vi "Initialize Dialog.vi"(8 "error in (no error)":errorcluster, 9 "SubPnl Refnum":refnum<vi>, 10 "VI Refnum":refnum<vi>, 11 "DataGrid Config Dialog in":refnum<class "DataGrid Config Dialog.lvclass">) -> (0 "error out":errorcluster, 1 "Data Type Selector Return":refnum<user-event>, 2 "Return Data":refnum<user-event>, 3 "DataGrid Config Dialog out":refnum<class "DataGrid Config Dialog.lvclass">)   [LabVIEW 2018, in "DataGrid Config Dialog.lvclass"]
uses:
  DataGrid Config Dialog.lvclass
  Data Type Classes/Generic/Generic Data Type.lvclass
  <vilib>/MGI/Panel Manager/Panel/Panel/Window/Dialog/Behavior.ctl
  DataGrid Config Dialog.lvclass/DataGrid Config Dialog.ctl
  <vilib>/MGI/Panel Manager/Panel/Panel/Subpanel/Subpanel.lvclass
  C:/Program Files (x86)/National Instruments/LabVIEW 2018/vi.lib/MGI/Panel Manager/Panel/Panel/Panel.lvclass
  <vilib>/MGI/Panel Manager/Panel/Panel/Window/Dialog/Dialog.lvclass
  <vilib>/MGI/Panel Manager/Panel/Panel/Subpanel/Subpanel.vi
  <vilib>/MGI/Panel Manager/Panel/Panel/Window/Dialog/Dialog.vi
  <vilib>/MGI/Panel Manager/Panel/Panel.lvlib
  <vilib>/MGI/Panel Manager/Panel/Panel/Panel.lvclass
  DataGrid Config/DataGrid Config.lvclass
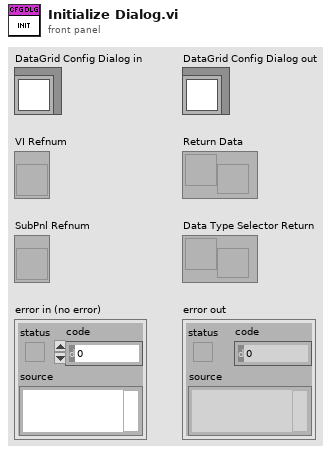
[diagram p1: front panel]
types:
  T1 = enum8{"Enabled", "Disabled", "Disabled and Grayed Out"}
  T2 = typedef "Panel.lvlib/Dialog.lvclass/Behavior.ctl" = enum32{"Floating", "Floating/Auto-Hide", "Modal"}
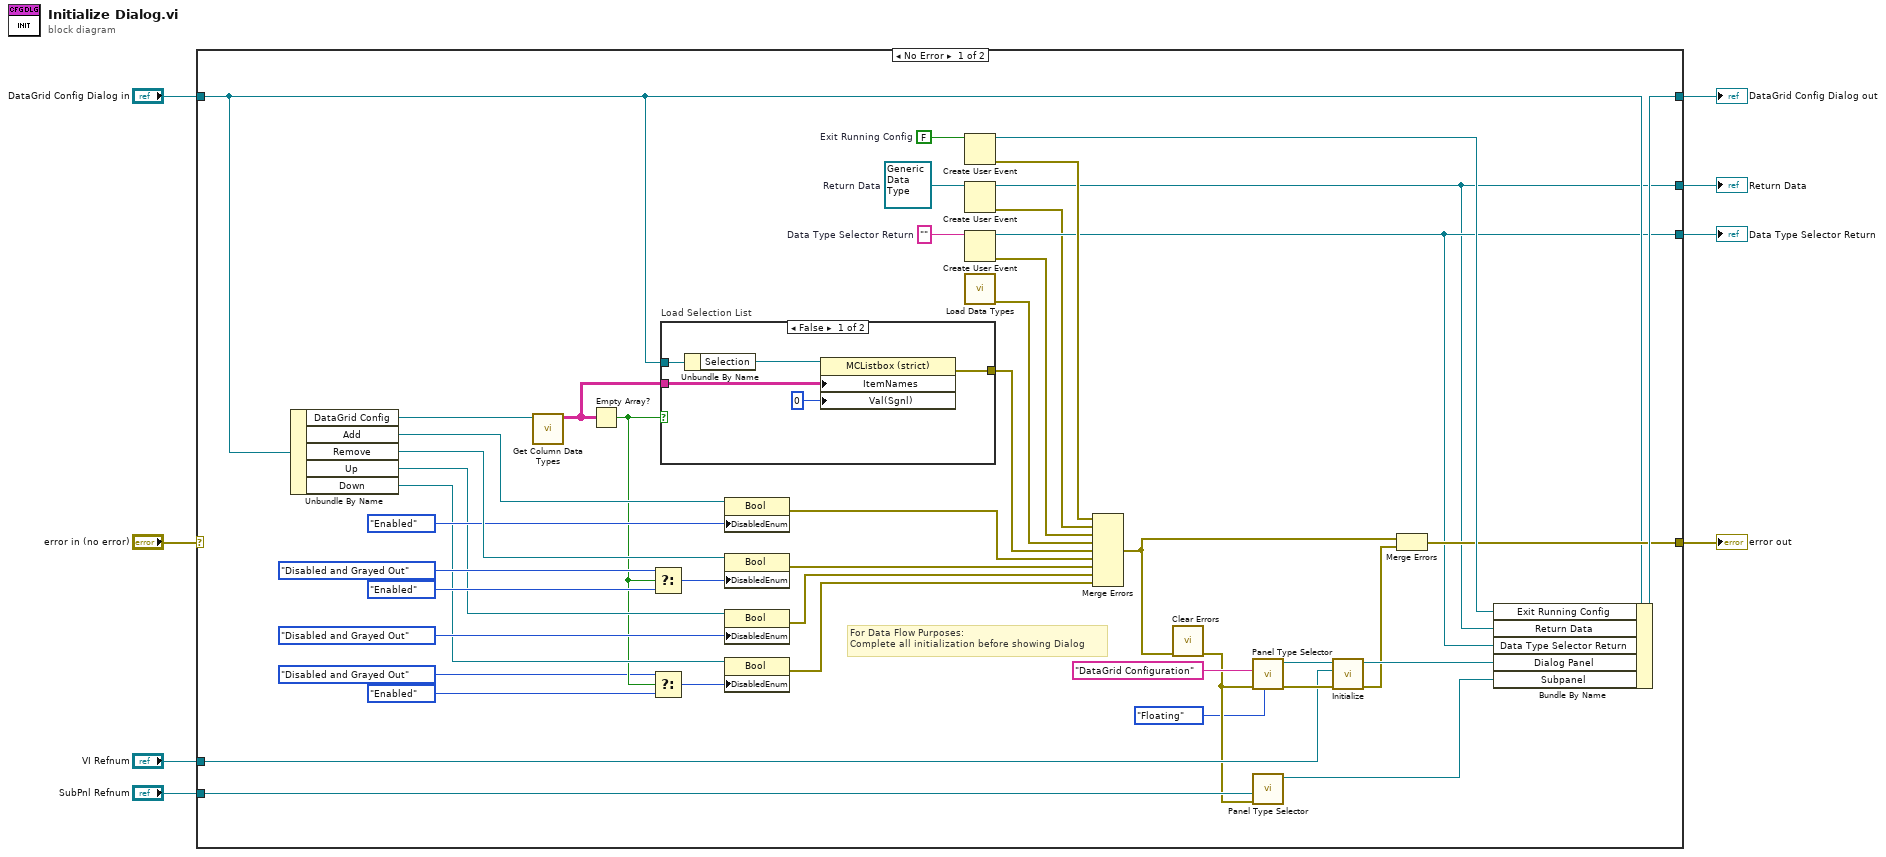
[diagram p0: block diagram]
diagram:
  n1 = case shown="No Error" "error in (no error)" {
    selector: "error in (no error)" -> [_ w59]
    tunnel: [w32 w59] -> w7
    tunnel: [w47 w58] -> w5
    tunnel: "DataGrid Config Dialog in" -> [w30 w58]
    tunnel: "VI Refnum" -> [w46 _]
    tunnel: "SubPnl Refnum" -> [w43 _]
    tunnel: [w20 _] -> w2
    tunnel: [w23 _] -> w1
    frame No Error {
      w25 = ""  # Data Type Selector Return
      w21 = refnum<class "Generic Data Type.lvclass"> refnum  # Return Data
      w49 = FALSE  # Exit Running Config
      # "For Data Flow Purposes:\nComplete all initialization before showing Dialog"
      n2 = Unbundle By Name(w30) -> ("DataGrid Config"=w45:refnum<class "DataGrid Config.lvclass">, "Add"=w39:refnum<vi>, "Remove"=w38:refnum<vi>, "Up"=w16:refnum<vi>, "Down"=w15:refnum<vi>)
      n3 = call "Get Column Data Types.vi"("DataGrid Config"=w45) -> ("Column Data Type Names"=w44:string[][])  [unwired: 10 in]
      n4 = Empty Array?(array=w44) -> (empty?=w14:bool)
      n5 = Select(t=T1."Disabled and Grayed Out" ("Disabled"), s=w14, f=T1."Enabled" ("Disabled")) -> (s? t:f=w27:T1)
      n6 = Select(t=T1."Disabled and Grayed Out" ("Disabled"), s=w14, f=T1."Enabled" ("Disabled")) -> (s? t:f=w11:T1)
      n7 = case "Load Selection List" shown="False" w14 {
        tunnel: w30 -> [w57 _]
        tunnel: [w55 _] -> w41
        tunnel: w44 -> [w54 _]
        frame False {
          n8 = Unbundle By Name(w57) -> ("Selection"=w56:refnum<vi>)
          n9 = property class="MCListbox (strict)"(reference=w56, "ItemNames"=w54, "Val(Sgnl)"=0 ("Value (Signaling)")) -> (error out=w55:errorcluster)  [unwired: 1 in, 1 out]
        }
        frame True {
        }
      }
      n10 = property class="Bool"(reference=w39, "DisabledEnum"=T1."Enabled" ("Disabled")) -> (error out=w37:errorcluster)  [unwired: 1 in, 1 out]
      n11 = property class="Bool"(reference=w38, "DisabledEnum"=w27) -> (error out=w36:errorcluster)  [unwired: 1 in, 1 out]
      n12 = property class="Bool"(reference=w16, "DisabledEnum"=T1."Disabled and Grayed Out" ("Disabled")) -> (error out=w10:errorcluster)  [unwired: 1 in, 1 out]
      n13 = property class="Bool"(reference=w15, "DisabledEnum"=w11) -> (error out=w9:errorcluster)  [unwired: 1 in, 1 out]
      n14 = Create User Event(user event datatype=w49) -> (user event=w35:refnum<user-event>, error out=w40:errorcluster)  [unwired: 1 in]
      n15 = Create User Event(user event datatype=w21) -> (user event=w20:refnum<user-event>, error out=w19:errorcluster)  [unwired: 1 in]
      n16 = Create User Event(user event datatype=w25) -> (user event=w23:refnum<user-event>, error out=w24:errorcluster)  [unwired: 1 in]
      n17 = call "Load Data Types.vi"() -> ("error out"=w22:errorcluster)  [unwired: 9 in, 2 out]
      n18 = Merge Errors(w40, w19, w24, w22, w41, w37, w36, w10, w9) -> (w34:errorcluster)
      n19 = call <vilib>:"Clear Errors.vi"("error in (no error)"=w34) -> ("error out"=w33:errorcluster)  [unwired: 5 in, 1 out]
      n20 = call-poly <vilib>:"Panel Type Selector.vi"("Behavior (Modal)"=Behavior."Floating", "Error In"=w33, "Default Title"="DataGrid Configuration") -> ("Error Out"=w52:errorcluster, "Dialog out"=w51:refnum<class "Dialog.lvclass">)  [unwired: 7 in]
      n21 = call-poly <vilib>:"Panel Type Selector.vi"("Error In"=w33, "Sub Panel"=w43) -> ("Subpanel Out"=w42:refnum<class "Subpanel.lvclass">)  [unwired: 8 in, 1 out]
      n22 = call <vilib>:"Initialize.vi"("error in (no error)"=w52, "VI Refnum"=w46, "Panel In"=w51) -> ("error out"=w31:errorcluster, "Panel Out"=w48:refnum<class "Dialog.lvclass">)  [unwired: 6 in, 1 out]
      n23 = Merge Errors(w34, w31) -> (w32:errorcluster)
      n24 = Bundle By Name(cluster=w30, "Exit Running Config"=w35, "Return Data"=w20, "Data Type Selector Return"=w23, "Dialog Panel"=w48, "Subpanel"=w42) -> (w47:refnum<class "DataGrid Config Dialog.lvclass">)
    }
    frame Error {
    }
  }
  "error out" <- w7
  "DataGrid Config Dialog out" <- w5
  "Return Data" <- w2
  "Data Type Selector Return" <- w1
